vi "Write.vi"(8 "error in (no error)":errorcluster, 10 "Voltage":dbl, 11 "Analog Output in":refnum<class "Analog Output.lvclass">) -> (0 "error out":errorcluster)   [LabVIEW 2021, in "Analog Output.lvlib" / "Analog Output.lvclass"]
uses:
  Analog Output.lvclass
  <vilib>/DAQmx/write.llb/DAQmx Write (Analog DBL 1Chan 1Samp).vi
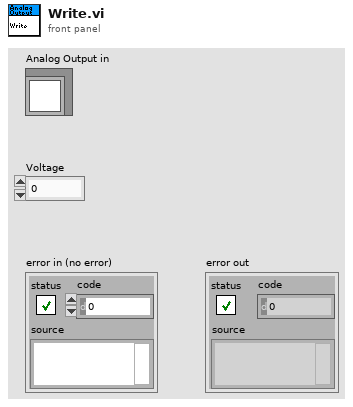
[diagram p1: front panel]
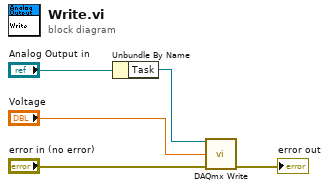
[diagram p0: block diagram]
diagram:
  n1 = Unbundle By Name("Analog Output in") -> ("Task"=w4:refnum<k21>)
  n2 = call-poly <vilib>:"DAQmx Write.vi"("task/channels in"=w4, "data"="Voltage", "error in"="error in (no error)") -> ("error out"=→"error out":errorcluster)  [unwired: 10 in, 2 out]
